vi "Anritsu VNA Calibrate.vi"(7 "Anritsu VNA":T5, 8 "error in (no error)":errorcluster, 10 "Parameters to Measure":T1[](array[typedef]) {"Channel" min=1 max=99 step=1; "Parameter"."Stimulus Port" min=1 step=1; "Parameter"."Response Port" min=1 step=1}, 11 "VISA Resource Name":refnum<visa-resource-name>) -> (0 "error out":errorcluster {"code" format="%.0x"}, 3 "dup VISA Resource Name":refnum<visa-resource-name>)   [LabVIEW 2011]
uses:
  TypeDefs/Anritsu VNA Instrument Info.ctl
  tests/S Parameter/TypeDefs/SP Parameter to Measure.ctl
  tests/S Parameter/TypeDefs/SP Parameter.ctl
  tests/S Parameter/TypeDefs/SP Calibration State.ctl
  tests/S Parameter/TypeDefs/SP Measurement Format.ctl
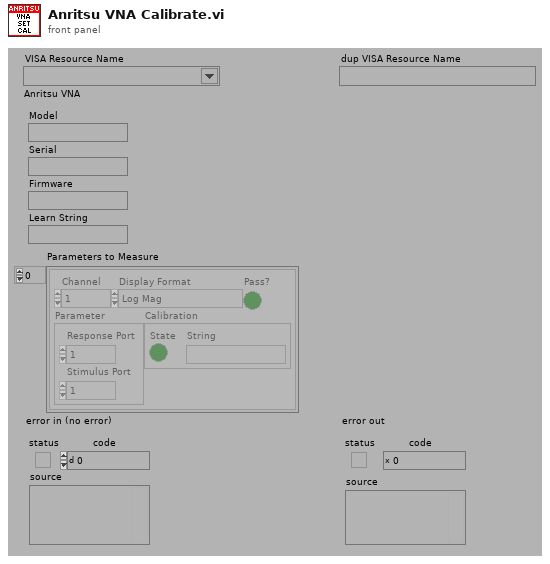
[diagram p1: front panel]
types:
  T1 = typedef "SP Parameter to Measure.ctl" = cluster{"Channel":i8, "Parameter":T2, "Calibration":T3, "Display Format":T4, "Pass?":bool}
  T2 = typedef "SP Parameter.ctl" = cluster{"Stimulus Port":i8, "Response Port":i8}
  T3 = typedef "SP Calibration State.ctl" = cluster{"State":bool, "String":string}
  T4 = typedef "SP Measurement Format.ctl" = enum32{"Log Mag", "Phase", "Delay", "Smith (R+jX)", "Polar (Re/Im)", "Linear Mag", "SWR", "Real", "Imaginary", "Smith (Lin/Phase)", "Smith (Log/Phase)", "Smith (Real/Imag)", "Smith (G+jB)", "Polar (Lin/Phase)", "Polar (Log/Phase)", "Expanded Phase", "Positive Phase", "Inverted Smith", "Unwrapped Phase", "Power Out", "Power In", "Linear Mag/Phase", "Log Mag/Phase", "Real/Imaginary"}
  T5 = typedef "Anritsu VNA Instrument Info.ctl" = cluster{"Model":string, "Serial":string, "Firmware":string, "Learn String":string}
  T6 = typedef "Anritsu VNA Model.ctl" = enum16{"Not Supported", "37XXXX", "MS20XXX", "MS462XX", "MS464XX"}
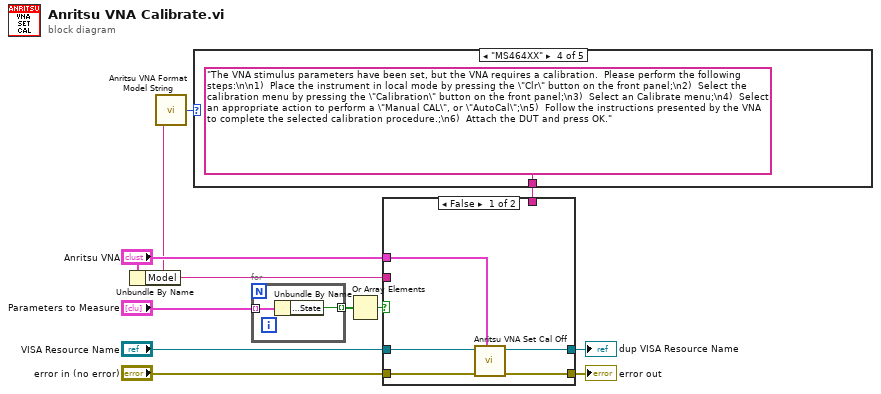
[diagram p0: block diagram]
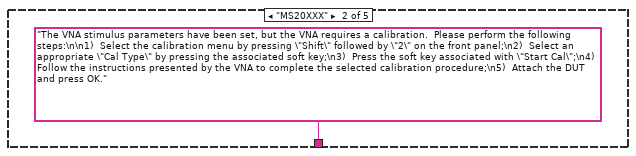
[diagram p3: hidden frame]
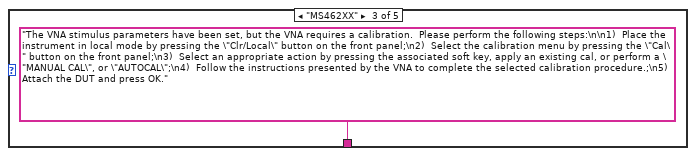
[diagram p4: hidden frame]
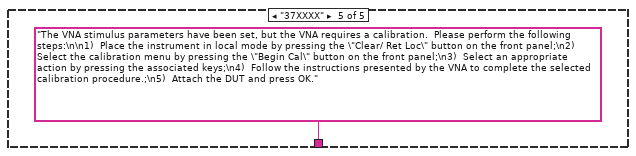
[diagram p5: hidden frame]
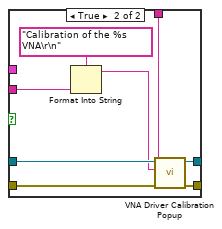
[diagram p6: hidden frame]
diagram:
  n1 = Unbundle By Name("Anritsu VNA") -> ("Model"=w2:string)
  n2 = call "Anritsu VNA Format Model String.vi"("Model"=w2) -> ("Model"=w1:T6)
  n3 = case shown="\"MS464XX\"" w1 {
    tunnel: [_ "The VNA stimulus parameters have been set, but the VNA requires a calibration.  Please perform the following steps:\n\n1)  Select the calibration menu by pressing \"Shift\" followed by \"2\" on the front panel;\n2)  Select an appropriate \"Cal Type\" by pressing the associated soft key;\n3)  Press the soft key associated with \"Start Cal\";\n4)  Follow the instructions presented by the VNA to complete the selected calibration procedure;\n5)  Attach the DUT and press OK." "The VNA stimulus parameters have been set, but the VNA requires a calibration.  Please perform the following steps:\n\n1)  Place the instrument in local mode by pressing the \"Clr/Local\" button on the front panel;\n2)  Select the calibration menu by pressing the \"Cal\" button on the front panel;\n3)  Select an appropriate action by pressing the associated soft key, apply an existing cal, or perform a \"MANUAL CAL\", or \"AUTOCAL\";\n4)  Follow the instructions presented by the VNA to complete the selected calibration procedure.;\n5)  Attach the DUT and press OK." "The VNA stimulus parameters have been set, but the VNA requires a calibration.  Please perform the following steps:\n\n1)  Place the instrument in local mode by pressing the \"Clr\" button on the front panel;\n2)  Select the calibration menu by pressing the \"Calibration\" button on the front panel;\n3)  Select an Calibrate menu;\n4)  Select an appropriate action to perform a \"Manual CAL\", or \"AutoCal\";\n5)  Follow the instructions presented by the VNA to complete the selected calibration procedure.;\n6)  Attach the DUT and press OK." "The VNA stimulus parameters have been set, but the VNA requires a calibration.  Please perform the following steps:\n\n1)  Place the instrument in local mode by pressing the \"Clear/ Ret Loc\" button on the front panel;\n2)  Select the calibration menu by pressing the \"Begin Cal\" button on the front panel;\n3)  Select an appropriate action by pressing the associated keys;\n4)  Follow the instructions presented by the VNA to complete the selected calibration procedure.;\n5)  Attach the DUT and press OK."] -> w4
    frame "Not Supported" {
    }
    frame "MS20XXX" {
    }
    frame "MS462XX" {
    }
    frame "MS464XX" {
    }
    frame "37XXXX" {
    }
  }
  n4 = for {
    tunnel: [w17] -> w6 mode=indexing
    tunnel: "Parameters to Measure" -> [w16] mode=indexing
    n5 = Unbundle By Name(w16) -> ("Calibration.State"=w17:bool)
  }
  n6 = Or Array Elements(Boolean array=w6) -> (logical OR=w7:bool)
  n7 = case shown="False" w7 {
    tunnel: "VISA Resource Name" -> [w18 w29]
    tunnel: "Anritsu VNA" -> [w22 _]
    tunnel: "error in (no error)" -> [w21 w26]
    tunnel: [w20 w25] -> w3
    tunnel: [w19 w29] -> w9
    tunnel: w2 -> [_ w27]
    tunnel: w4 -> [_ w24]
    frame False {
      n8 = call "Anritsu VNA Set Cal Off.vi"("Anritsu VNA"=w22, "error in (no error)"=w21, "VISA Resource Name"=w18) -> ("error out"=w20:errorcluster, "dup VISA Resource Name"=w19:refnum<visa-resource-name>)  [unwired: 7 out]
    }
    frame True {
      n9 = Format Into String(format string="Calibration of the %s VNA\r\n", w27) -> (resulting string=w23:string)  [unwired: 2 in, 1 out]
      n10 = call "VNA Driver Calibration Popup.vi"("error in (no error)"=w26, "RequestedCal"=w23, "Message (\"\")"=w24) -> ("error out"=w25:errorcluster)  [unwired: 8 out]
    }
  }
  "error out" <- w3
  "dup VISA Resource Name" <- w9
